vi "Set Discovery Info.vi"(8 "error in (no error)":errorcluster, 10 "Discovery Info":T1, 11 "Node in":refnum<class "Node.lvclass">) -> (0 "error out":errorcluster, 3 "Node out":refnum<class "Node.lvclass">)   [LabVIEW 2020, in "Vecto.lvlib" / "Node.lvclass"]
uses:
  Node.lvclass
  Discovery Info.ctl
  Node.lvclass/Node.ctl
  Vecto.lvlib
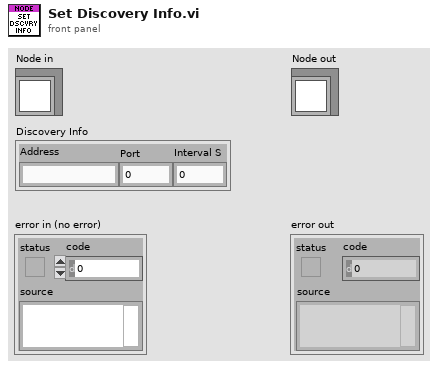
[diagram p1: front panel]
types:
  T1 = typedef "Vecto.lvlib/Discovery Info.ctl" = cluster{"Address":string, "Port":u16, "Interval S":dbl}
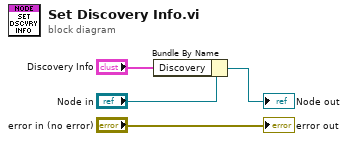
[diagram p0: block diagram]
diagram:
  n1 = Bundle By Name(cluster="Node in", "Discovery"="Discovery Info") -> (→"Node out":refnum<class "Node.lvclass">)
  "error out" <- "error in (no error)"
